vi "Climb Controller.vi"(8 "error in":errorcluster) -> ()   [LabVIEW 2018]
doc: "This VI executes continuously carrying out the current operation and responding to updates or new operations. It will often contain the timing or control code that is difficult to place directly in TeleOp. This VI generally opens all sensors and motors and isolates the rest of the robot code from knowing how the operations are carried out."
uses:
  <vilib>/Rock Robotics/WPI/Framework/Completion Status.ctl
  Climb Setpoints.ctl
  Climb Operations.ctl
  <vilib>/Rock Robotics/SystemInterfaces/DIO/FPGA_DIOChannel.ctl
  <vilib>/Rock Robotics/WPI/ThirdParty/Phoenix-LabVIEW/Motor Controller/Controls/CTRE_Phoenix_MotorControl_FeedbackDevice.ctl
  <vilib>/Rock Robotics/WPI/ThirdParty/REV Robotics/SPARK MAX/Typedef/Spark MAX Control Type.ctl
  <vilib>/Rock Robotics/WPI/ThirdParty/Phoenix-LabVIEW/Motor Controller/Controls/CTRE_Phoenix_MotorControl_ControlMode.ctl
  <vilib>/Rock Robotics/WPI/Switch/WPI_SwitchOpenLimit.vi
  <vilib>/Rock Robotics/WPI/ThirdParty/Phoenix-LabVIEW/Motor Controller/Get/CTRE_Phoenix_MotorController_GetQuadratureData.vi
  <vilib>/Rock Robotics/Network Tables/NT Write Number.vi
  <vilib>/Rock Robotics/Network Tables/NT Write Boolean.vi
  ADIS16448 IMU/ADIS16448_IMU.lvlib
panel:
  in  "Offset Lv 2":dbl=19.75
  in  "Initilization 2":dbl=17.0 format="%#_13g"
  out "IPCed":dbl
  in  "Interactive Values":T1={"Operation"=enum."Read Current", "Setpoint Rhino"=0.0, "Setpoint WHEELS"=0.0, "Roll"=0.0, "Pitch"=0.0, "Reset"=FALSE, "Speedy Tilt"={"Right"=TRUE, "Left"=TRUE}, "Climb"=enum."Level 1-3", "New Pos?"=FALSE, "Defense mode?"=FALSE}
  out "Current\nCmd":string
  in  "Buttons":cluster{"Execute Cmd":bool, "Abort Cmd":bool}
  out "Command Timing":cluster{"Start Time (ms)":u32, "Iterations":i32}
  out "Status":T3
  # "Tip: It may be helpful to observe inputs and sensor values.\nYou may also want to display tuning or debugging controls."
  # "Interactive Command: You may fill in the settings for a command\nand schedule it with the Execute button. You can observe and abort\nany command while fine tuning the code for the controller."
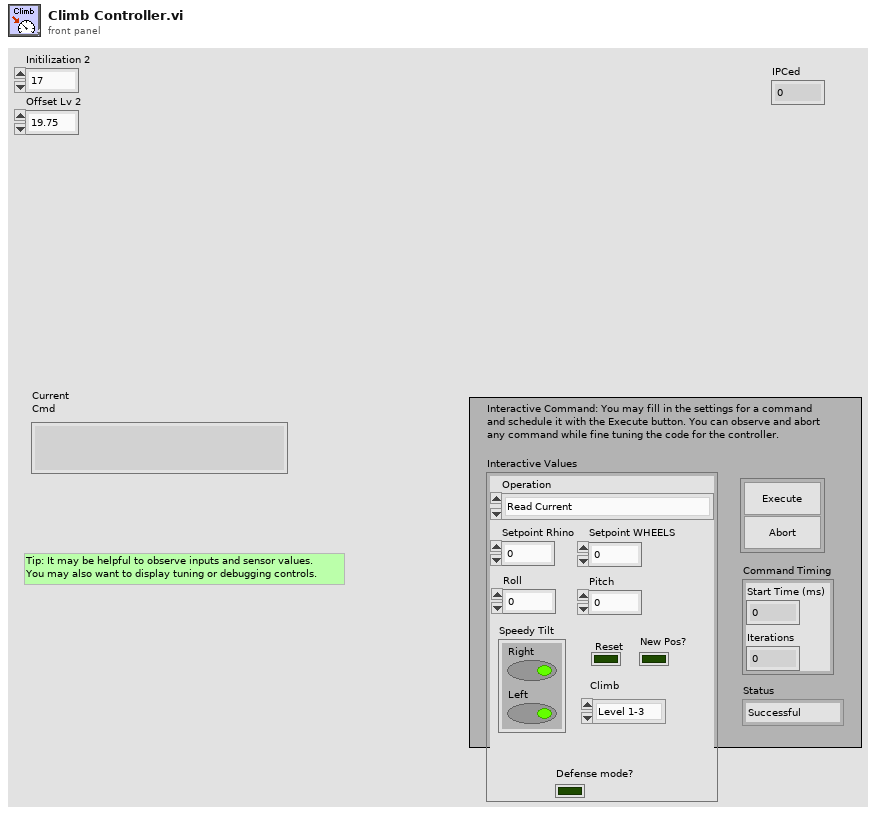
[diagram p1: front panel]
types:
  T1 = typedef "Climb Setpoints.ctl" = cluster{"Operation":T2, "Setpoint Rhino":dbl, "Setpoint WHEELS":dbl, "Roll":dbl, "Pitch":dbl, "Reset":bool, "Speedy Tilt":cluster{"Right":bool, "Left":bool}, "Climb":enum16{"Level 1-3", "Level 1-2", "Level 2-3"}, "New Pos?":bool, "Defense mode?":bool}
  T2 = typedef "Climb Operations.ctl" = enum16{"Reserve", "Read Current", "Immediate", "Ready", "Auto-Climb", "Reset/Turbo-Tilt", "Manual Climb"}
  T3 = typedef "Completion Status.ctl" = enum16{"Successful", "Aborted", "Incomplete"}
  T4 = cluster{"P Gain":dbl, "I Gain":dbl, "D Gain":dbl, "F Gain":dbl, "I Zone":dbl, "Min Output":dbl, "Max Output":dbl}
  T5 = typedef "CTRE_Phoenix_MotorControl_FeedbackDevice.ctl" = i8
  T6 = typedef "FPGA_DIOChannel.ctl" = enum8{"DIO 0", "DIO 1", "DIO 2", "DIO 3", "DIO 4", "DIO 5", "DIO 6", "DIO 7", "DIO 8", "DIO 9", "DIO MXP 0", "DIO MXP 1", "DIO MXP 2", "DIO MXP 3", "DIO MXP 4", "DIO MXP 5", "DIO MXP 6", "DIO MXP 7", "DIO MXP 8", "DIO MXP 9", "DIO MXP 10", "DIO MXP 11", "DIO MXP 12", "DIO MXP 13", "DIO MXP 14", "DIO MXP 15", "SPI Port CS1", "SPI Port CS2", "SPI Port CS3", "SPI Port MISO", "SPI Port MOSI", "Invalid"}
  T7 = typedef "WPI_MotorControlDeviceRef.ctl" = cluster{"DeviceStatus":errorcluster, "Type":T8, "PWM":cluster{"PWM Channel":T9, "DeadBand":T10}, "CAN":cluster{"Device Number":u8, "SetOutput VI Ref":variant, "GetOutput VI Ref":variant, "Enable VI Ref":variant, "Disable VI Ref":variant, "Data":variant}, "Invert":bool, "DIO PWM":cluster{"PWM \"Enable\" Channel":T9, "DIOChannel":T6, "PWM Rate":dbl}}
  T8 = typedef "WPI_MotorControlType.ctl" = enum16{"PWM", "CAN", "DIO PWM"}
  T9 = typedef "FPGA_DIOPWMChannel.ctl" = enum8{"PWM 0", "PWM 1", "PWM 2", "PWM 3", "PWM 4", "PWM 5", "PWM 6", "PWM 7", "PWM 8", "PWM 9", "PWM MXP 0", "PWM MXP 1", "PWM MXP 2", "PWM MXP 3", "PWM MXP 4", "PWM MXP 5", "PWM MXP 6", "PWM MXP 7", "PWM MXP 8", "PWM MXP 9", "Invalid"}
  T10 = typedef "WPI_PWMDeadband.ctl" = cluster{"Name":string, "maxPositivePwm":i32, "minPositivePwm":i32, "centerPwm":i32, "maxNegativePwm":i32, "minNegativePwm":i32, "angularRange":u16}
  T11 = typedef "WPI_SwitchDevRef.ctl" = cluster{"DevStatus":errorcluster, "DIO Channel":T6, "CntIndex":T12, "Normally Closed":bool}
  T12 = typedef "FPGA_CounterCtrSystemIndex.ctl" = enum8{"Ctr 0", "Ctr 1", "Ctr 2", "Ctr 3", "Ctr 4", "Ctr 5", "Ctr 6", "Ctr 7", "Invalid"}
  T13 = typedef "Command Status Info.ctl" = cluster{"Name":string, "Status":T3, "notifier out":T14}
  T14 = typedef "Completion Notifier.ctl" = refnum<notifier>
  T15 = cluster{"Current Command":T1, "Command Timing":cluster{"Start Time (ms)":u32, "Iterations":i32}, "Command Arguments":cluster{"Command Info":T13, "Description":string, "Default Command":T1, "queue out":refnum<queue>, "Subsystem Name":string}}
  T16 = typedef "ADIS16448_IMU.lvlib/ADI_IMU_ADIS16448_IMUDevRef.ctl" = cluster{"DevStatus":errorcluster, "Handle":i32, "SPI Bus":T17, "Device Found":bool, "Device Ready":bool, "Yaw Axis":enum16{"X", "Y", "Z"}, "AHRS Algorithm":enum16{"Complementary", "Madgwick"}, "Serial":u16, "Lot ID 2":u16, "Lot ID 1":u16, "Bytes Per Sample":u16, "Calibrate On Open?":bool}
  T17 = typedef "spi_bus.ctl" = enum16{"SPI On-Board, CS0", "SPI On-Board, CS1", "SPI On-Board, CS2", "SPI On-Board, CS3", "SPI MXP", "Invalid"}
  T18 = typedef "Spark MAX Control Type.ctl" = enum16{"Percent VBus", "Voltage", "Velocity", "Position", "Smart Motion", "Current", "Smart Velocity"}
  T19 = typedef "CTRE_Phoenix_MotorControl_ControlMode.ctl" = u16
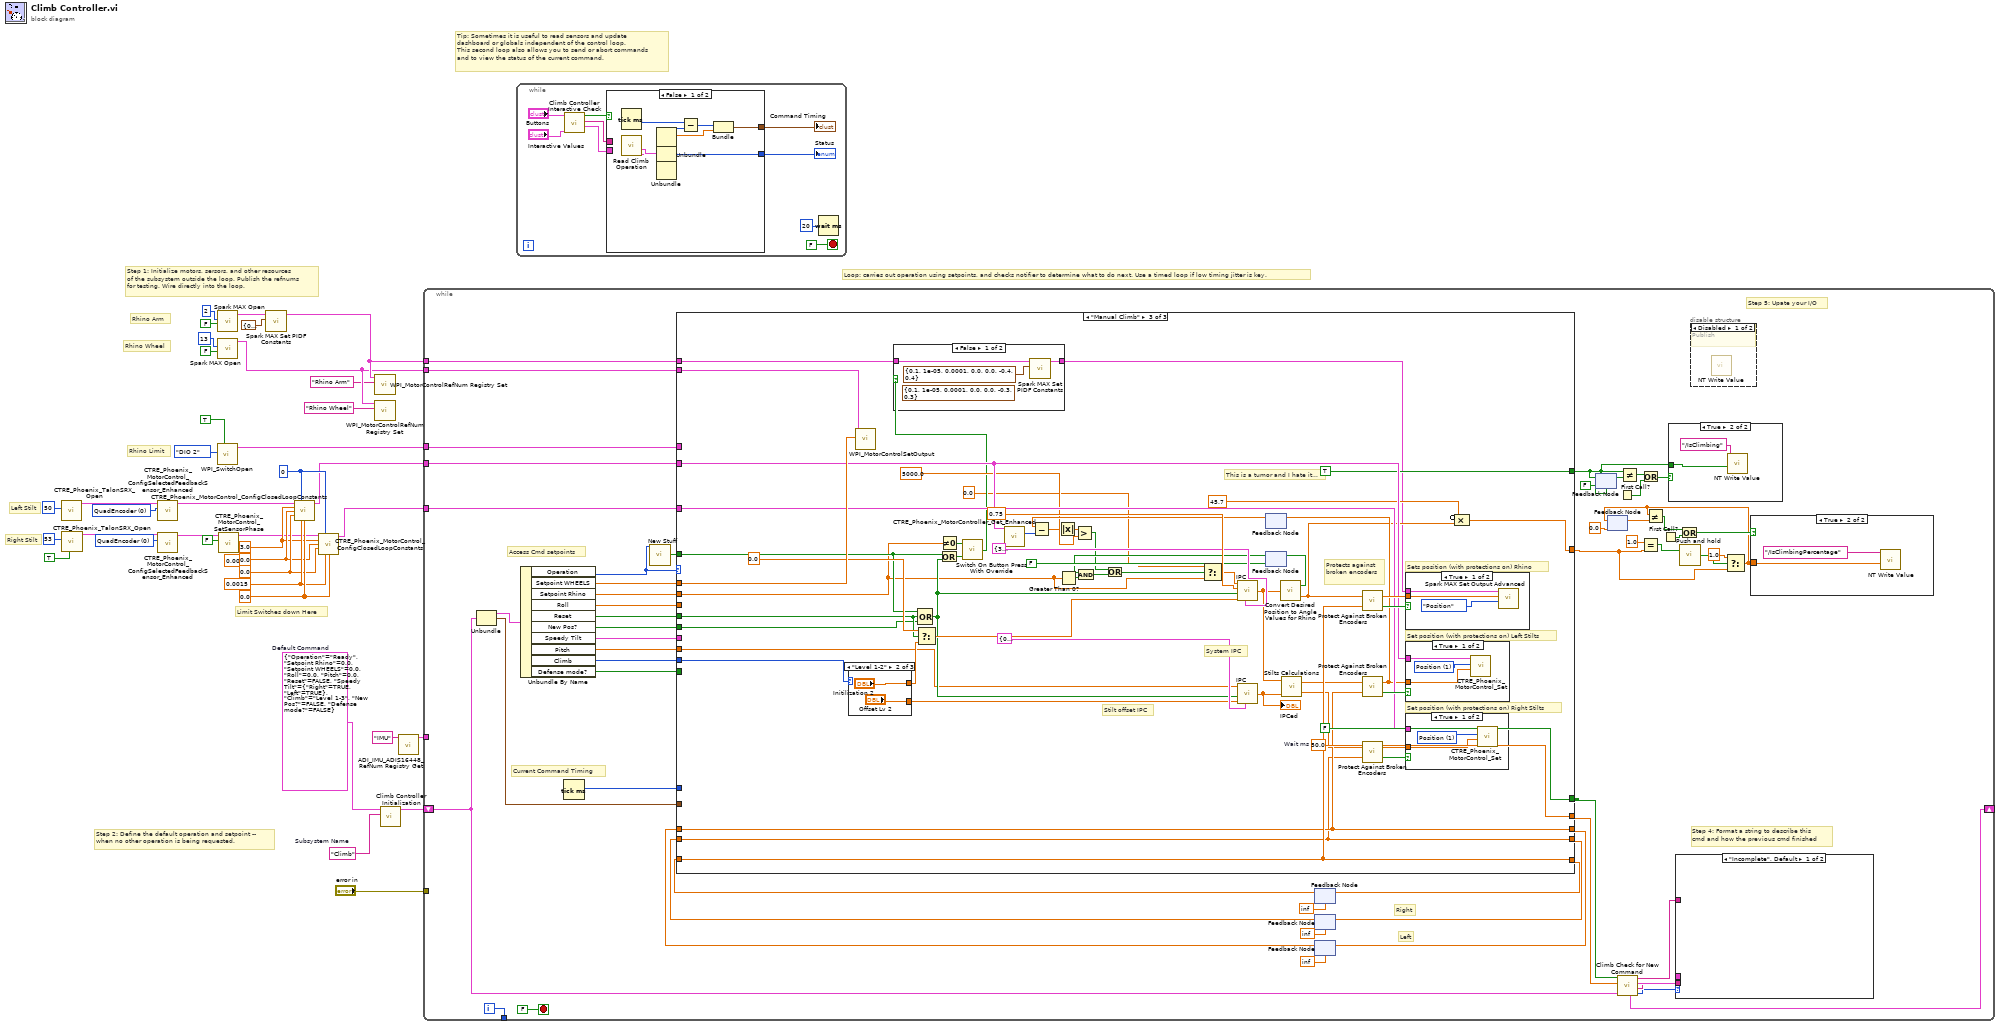
[diagram p0: block diagram]
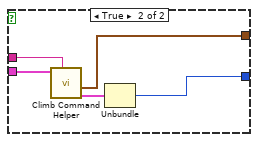
[diagram p2: hidden frame]
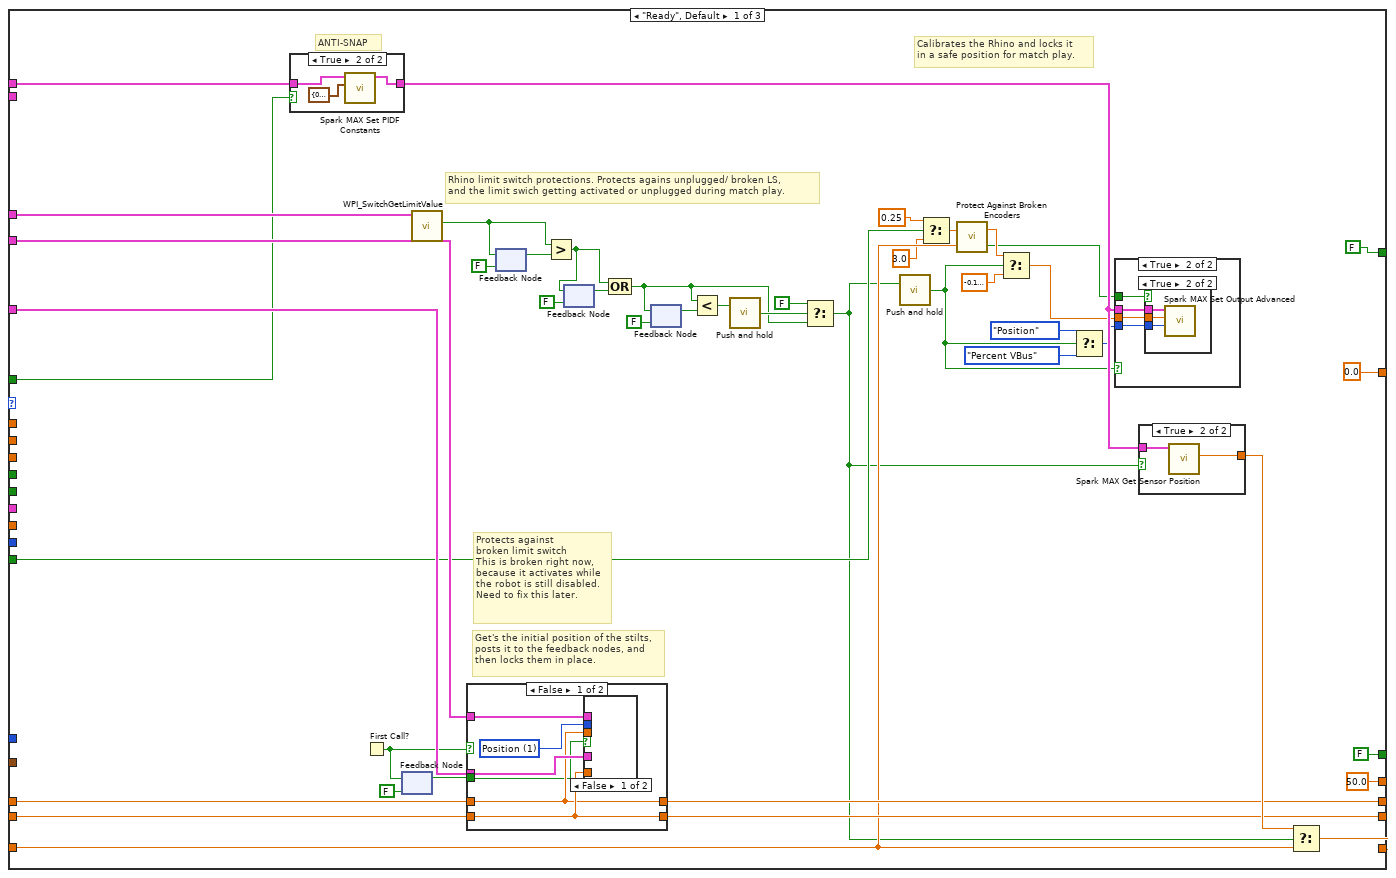
[diagram p5: hidden frame]
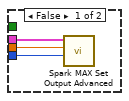
[diagram p6: hidden frame]
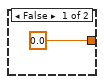
[diagram p9: hidden frame]
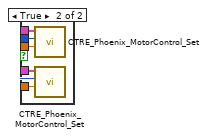
[diagram p10: hidden frame]
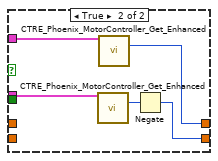
[diagram p11: hidden frame]
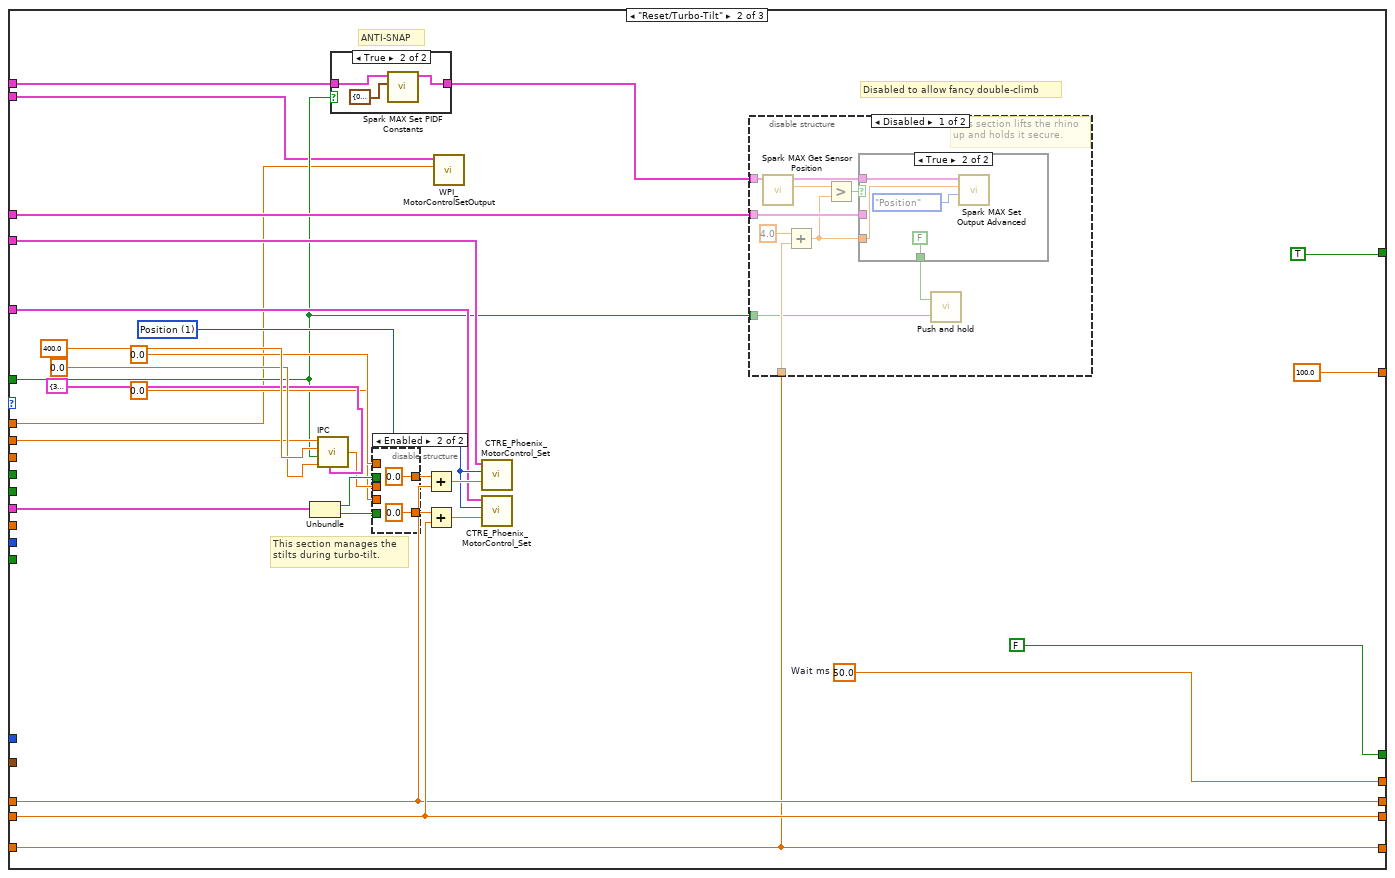
[diagram p12: hidden frame]
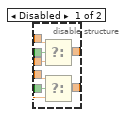
[diagram p13: hidden frame]
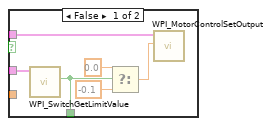
[diagram p14: hidden frame]
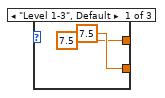
[diagram p17: hidden frame]
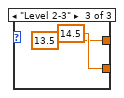
[diagram p18: hidden frame]
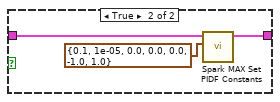
[diagram p19: hidden frame]
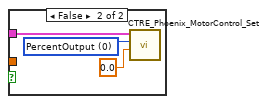
[diagram p20: hidden frame]
diagram:
  (unwired) 0.0001 ("I")
  w16 = 0.0015 ("F")
  w15 = 0.0 ("D")
  w14 = 0.0 ("I")
  w13 = 3.0 ("P")
  w17 = 0.0 ("I Zone")
  w12 = 0 ("slotIdx")
  w24 = T5 0 items=["QuadEncoder"=0, "Analog"=2, "Tachometer"=4, "Pulse Width Encoded Position"=8, "Sensor Sum (S0 + S1)"=9, "Sensor Difference (D0 - D1)"=10, "Remote Source 0"=11, "Remote Source 1"=12, "Software Emulated"=15] ("Feedback Device")
  w25 = T5 0 items=["QuadEncoder"=0, "Analog"=2, "Tachometer"=4, "Pulse Width Encoded Position"=8, "Sensor Sum (S0 + S1)"=9, "Sensor Difference (D0 - D1)"=10, "Remote Source 0"=11, "Remote Source 1"=12, "Software Emulated"=15] ("Feedback Device")
  w5 = T1 {"Operation"=enum."Ready", "Setpoint Rhino"=0.0, "Setpoint WHEELS"=0.0, "Roll"=0.0, "Pitch"=0.0, "Reset"=FALSE, "Speedy Tilt"={"Right"=TRUE, "Left"=TRUE}, "Climb"=enum."Level 1-3", "New Pos?"=FALSE, "Defense mode?"=FALSE}  # Default Command
  w36 = "Climb"  # Subsystem Name
  # "Limit Switches down Here"
  # "Left Stilt"
  # "Rhino Limit"
  # "Right Stilt"
  # "Rhino Wheel"
  # "Rhino Arm"
  # "Tip: Sometimes it is useful to read sensors and update\ndashboard or globals independent of the control loop.\nThis second loop also allows you to send or abort commands\nand to view the status of the current command."
  # "Step 2: Define the default operation and setpoint --\nwhen no other operation is being requested."
  # "Step 1: Initialize motors, sersors, and other resources\nof the subsystem outside the loop. Publish the refnums\nfor testing. Wire directly into the loop."
  # "Loop: carries out operation using setpoints, and checks notifier to determine what to do next. Use a timed loop if low timing jitter is key."
  n1 = call <vilib>:"CTRE_Phoenix_TalonSRX_Open.vi"("Device Number"=u8 50) -> ("CAN Talon SRX Ref"=w23:T7)  [unwired: 9 in, 1 out]
  n2 = call <vilib>:"CTRE_Phoenix_TalonSRX_Open.vi"("Invert"=TRUE, "Device Number"=u8 53) -> ("CAN Talon SRX Ref"=w22:T7)  [unwired: 8 in, 1 out]
  n3 = call <vilib>:"CTRE_Phoenix_MotorControl_ConfigSelectedFeedbackSensor_Enhanced.vi"("Feedback Device"=w24, "PhoenixMotorControlDevRef"=w23) -> ("PhoenixMotorControlDevRef"=w11:T7)  [unwired: 8 in, 1 out]
  n4 = call <vilib>:"CTRE_Phoenix_MotorControl_ConfigSelectedFeedbackSensor_Enhanced.vi"("Feedback Device"=w25, "PhoenixMotorControlDevRef"=w22) -> ("PhoenixMotorControlDevRef"=w21:T7)  [unwired: 8 in, 1 out]
  n5 = call-poly <vilib>:"WPI_SwitchOpen.vi"("Normally Closed"=TRUE, "DIO Channel"=FPGA_DIOChannel."DIO 2") -> ("SwitchDevRef"=w27:T11)  [unwired: 8 in, 1 out]
  n6 = call <vilib>:"Spark MAX Open.vi"("Invert"=FALSE, "Device Number"=u8 2) -> ("MotorControlDeviceRef"=w18:T7)  [unwired: 8 in, 1 out]
  n7 = call <vilib>:"Spark MAX Open.vi"("Invert"=FALSE, "Device Number"=u8 13) -> ("MotorControlDeviceRef"=w3:T7)  [unwired: 8 in, 1 out]
  n8 = call <vilib>:"CTRE_Phoenix_MotorControl_SetSensorPhase.vi"("PhaseSensor"=FALSE, "PhoenixMotorControlDevRef"=w21) -> ("PhoenixMotorControlDevRef"=w10:T7)  [unwired: 8 in, 1 out]
  n9 = call <vilib>:"Spark MAX Set PIDF Constants.vi"("PID Constants"=T4 {"P Gain"=0.1, "I Gain"=1e-05, "D Gain"=0.0, "F Gain"=0.0, "I Zone"=0.0, "Min Output"=-1.0, "Max Output"=1.0}, "MotorControlDeviceRef"=w18) -> ("MotorControlDeviceRef"=w4:T7)  [unwired: 8 in, 1 out]
  n10 = call <vilib>:"CTRE_Phoenix_MotorControl_ConfigClosedLoopConstants.vi"("PhoenixMotorControlDevRef"=w11, "slotIdx"=w12, "P"=w13, "I"=w14, "D"=w15, "F"=w16, "I Zone"=w17) -> ("PhoenixMotorControlDevRef"=w7:T7)  [unwired: 7 in, 1 out]
  n11 = call <vilib>:"CTRE_Phoenix_MotorControl_ConfigClosedLoopConstants.vi"("PhoenixMotorControlDevRef"=w10, "slotIdx"=w12, "P"=w13, "I"=w14, "D"=w15, "F"=w16, "I Zone"=w17) -> ("PhoenixMotorControlDevRef"=w6:T7)  [unwired: 7 in, 1 out]
  n12 = call <vilib>:"WPI_MotorControlRefNum Registry Set.vi"("refnum name"="Rhino Arm", "MotorControlDevRef"=w4) -> ()  [unwired: 8 in, 2 out]
  n13 = call <vilib>:"WPI_MotorControlRefNum Registry Set.vi"("refnum name"="Rhino Wheel", "MotorControlDevRef"=w3) -> ()  [unwired: 8 in, 2 out]
  n14 = call "Climb Controller Initialization.vi"("Subsystem Name"=w36, "Default Command"=w5) -> ("Current Command"=w37:T15)  [unwired: 9 in]
  n15 = call "ADI_IMU_ADIS16448_RefNum Registry Get.vi"("refnum name"="IMU") -> ("ADI IMU DevRef"=w9:T16)  [unwired: 9 in, 1 out]
  n16 = while {
    shift-right: [w88] -> _
    shift-left: w37 -> [w81]
    tunnel: [w92] -> _
    tunnel: "error in" -> [_]
    tunnel: w27 -> [w80]
    tunnel: w4 -> [w76]
    tunnel: w3 -> [w75]
    tunnel: w7 -> [w63]
    tunnel: w6 -> [w62]
    tunnel: w9 -> [_]
    i -> [w92]
    stop <- FALSE stop-if-true
    # "Right"
    # "Left"
    # "Step 5: Upate your I/O"
    # "Step 4: Format a string to describe this\ncmd and how the previous cmd finished"
    # "Current Command Timing"
    # "Access Cmd setpoints"
    n17 = Unbundle(w81) -> ("Current Command"=w91:T1, "Command Timing"=w89:cluster{"Start Time (ms)":u32, "Iterations":i32})  [unwired: 1 out]
    n18 = Unbundle By Name(w91) -> ("Operation"=w61:T2, "Setpoint WHEELS"=w58:dbl, "Setpoint Rhino"=w57:dbl, "Roll"=w68:dbl, "Reset"=w67:bool, "New Pos?"=w66:bool, "Speedy Tilt"=w65:cluster{"Right":bool, "Left":bool}, "Pitch"=w64:dbl, "Climb"=w59:enum16{"Level 1-3", "Level 1-2", "Level 2-3"}, "Defense mode?"=w56:bool)
    n19 = Tick Count (ms)() -> (millisecond timer value=w90:u32)
    n20 = call "New Stuff.vi"("Variant"=w61) -> ("x != y?"=w60:bool)  [unwired: 26 in]
    n21 = feedback #1(inf) -> (w78:dbl)
    n22 = feedback #2(inf) -> (w72:dbl)
    n23 = feedback #3(inf) -> (w71:dbl)
    n24 = case shown="\"Manual Climb\"" w61 {
      tunnel: [50.0 ("Wait ms") w184 w288] -> w86
      tunnel: [FALSE ("Output") FALSE ("Output") FALSE] -> w87
      tunnel: w89 -> [_ _ _]
      tunnel: w57 -> [_ w193 w244]
      tunnel: w90 -> [_ _ _]
      tunnel: w80 -> [w142 w199 _]
      tunnel: [w140 w197 w285] -> w79
      tunnel: w78 -> [w133 w197 w285]
      tunnel: w58 -> [_ w178 w289]
      tunnel: w76 -> [w129 w183 w270]
      tunnel: w75 -> [_ w179 w290]
      tunnel: w63 -> [w135 w195 w275]
      tunnel: w62 -> [w134 w194 w277]
      tunnel: w72 -> [w136 w200 w278]
      tunnel: w71 -> [w137 w198 w282]
      tunnel: [w138 w200 w278] -> w70
      tunnel: [w139 w198 w282] -> w69
      tunnel: w68 -> [_ _ _]
      tunnel: w67 -> [_ _ w247]
      tunnel: w66 -> [_ _ w246]
      tunnel: w65 -> [_ w192 _]
      tunnel: w64 -> [_ _ w245]
      tunnel: w60 -> [w128 w181 w257]
      tunnel: w59 -> [_ _ w248]
      tunnel: w56 -> [w125 _ _]
      tunnel: [FALSE ("Assisted?") TRUE ("Assisted?") TRUE ("Assisted?")] -> w47
      tunnel: [0.0 ("t") 100.0 ("t") w241] -> w41
      frame "Ready", Default {
        # "Rhino limit switch protections. Protects agains unplugged/ broken LS,\nand the limit swich getting activated or unplugged during match play."
        # "Protects against\nbroken limit switch\nThis is broken right now,\nbecause it activates while\nthe robot is still disabled. \nNeed to fix this later."
        # "Calibrates the Rhino and locks it\nin a safe position for match play."
        # "Get's the initial position of the stilts,\nposts it to the feedback nodes, and\nthen locks them in place."
        # "ANTI-SNAP"
        n25 = case shown="True" w128 {
          tunnel: w129 -> [w153 w155]
          tunnel: [w153 w154] -> w124
          frame False {
          }
          frame True {
            n26 = call <vilib>:"Spark MAX Set PIDF Constants.vi"("PID Constants"=T4 {"P Gain"=0.1, "I Gain"=1e-05, "D Gain"=0.0001, "F Gain"=0.0, "I Zone"=0.0, "Min Output"=-0.3, "Max Output"=0.3}, "MotorControlDeviceRef"=w155) -> ("MotorControlDeviceRef"=w154:T7)  [unwired: 8 in, 1 out]
          }
        }
        n27 = First Call?() -> (First Call?: T/F=w132:bool)
        n28 = feedback #4(FALSE ("First Call?: T/F")) -> (w130:bool)
        n29 = feedback-in #4(w132) -> ()
        n30 = call <vilib>:"WPI_SwitchGetLimitValue.vi"("SwitchDevRef"=w142) -> ("Switch Pressed"=w109:bool)  [unwired: 8 in, 2 out]
        n31 = case shown="False" w132 {
          tunnel: w135 -> [w165 w175]
          tunnel: w134 -> [w164 w174]
          tunnel: [w161 w173] -> w139
          tunnel: [w162 w171] -> w138
          tunnel: w137 -> [w161 _]
          tunnel: w136 -> [w162 _]
          tunnel: w130 -> [w160 _]
          frame False {
            w163 = T19 1 items=["PercentOutput"=0, "Position"=1, "Velocity"=2, "Current"=3, "Follower"=5, "MotionProfile"=6, "MotionMagic"=7, "MotionProfileArc"=10, "Disabled"=15] ("Control Mode")
            n32 = case shown="False" w160 {
              tunnel: w165 -> [_ w170]
              tunnel: w164 -> [_ w169]
              tunnel: w163 -> [_ w168]
              tunnel: w162 -> [_ w167]
              tunnel: w161 -> [_ w166]
              frame False {
              }
              frame True {
                n33 = call <vilib>:"CTRE_Phoenix_MotorControl_Set.vi"("Output"=w166, "Control Mode"=w168, "PhoenixMotorControlDevRef"=w170) -> ()  [unwired: 7 in, 2 out]
                n34 = call <vilib>:"CTRE_Phoenix_MotorControl_Set.vi"("Output"=w167, "Control Mode"=w168, "PhoenixMotorControlDevRef"=w169) -> ()  [unwired: 7 in, 2 out]
              }
            }
          }
          frame True {
            n35 = call-poly <vilib>:"CTRE_Phoenix_MotorController_Get_Enhanced.vi"("PhoenixMotorControlDevRef"=w174) -> ("Quadrature Position"=w172:i32)  [unwired: 11 in, 3 out]
            n36 = call-poly <vilib>:"CTRE_Phoenix_MotorController_Get_Enhanced.vi"("PhoenixMotorControlDevRef"=w175) -> ("Quadrature Position"=w173:i32)  [unwired: 11 in, 3 out]
            n37 = Negate(x=w172) -> (-x=w171:i32)
          }
        }
        n38 = feedback-in #5(w109) -> ()
        n39 = feedback #5(FALSE ("Switch Pressed")) -> (w110:bool)
        n40 = Greater?(x=w109, y=w110) -> (0:w106:bool)
        n41 = feedback #6(FALSE ("Switch Pressed")) -> (w105:bool)
        n42 = feedback-in #6(w106) -> ()
        n43 = Compound Arithmetic op=OR(w106, w105) -> (w100:bool)
        n44 = feedback-in #7(w100) -> ()
        n45 = feedback #7(FALSE) -> (w103:bool)
        n46 = Less?(x=w100, y=w103) -> (x < y?=w102:bool)
        n47 = call "Push and hold.vi"("Input"=w102) -> ("Output"=w101:bool)  [unwired: 1 in]
        n48 = Select(t=FALSE, s=w101, f=w100) -> (s? t:f=w98:bool)
        n49 = call "Push and hold.vi"("Input"=w98) -> ("Output"=w111:bool)  [unwired: 1 in]
        n50 = Select(t=0.25, s=w125, f=3.0 ("t")) -> (s? t:f=w114:dbl)
        n51 = call "Protect Against Broken Encoders.vi"("Rhino Offset"=w133, "Output"=w114) -> ("Boolean"=w115:bool, "Numeric"=w118:dbl)
        n52 = Select(t=w118, s=w111, f=-0.10000000000000003) -> (s? t:f=w117:dbl)
        n53 = Select(t=Spark_MAX_Control_Type."Position" ("Control Mode"), s=w111, f=Spark_MAX_Control_Type."Percent VBus" ("Control Mode")) -> (s? t:f=w116:T18)
        n54 = case shown="True" w111 {
          tunnel: w117 -> [w144 w149]
          tunnel: w116 -> [w143 w148]
          tunnel: w124 -> [w145 w147]
          tunnel: w115 -> [_ w146]
          frame False {
            n55 = call <vilib>:"Spark MAX Set Output Advanced.vi"("Control Mode"=w143, "Setpoint"=w144, "MotorControlDevRef"=w145) -> ()  [unwired: 7 in, 2 out]
          }
          frame True {
            n56 = case shown="True" w146 {
              tunnel: w149 -> [_ w152]
              tunnel: w148 -> [_ w151]
              tunnel: w147 -> [_ w150]
              frame False {
              }
              frame True {
                n57 = call <vilib>:"Spark MAX Set Output Advanced.vi"("Control Mode"=w151, "Setpoint"=w152, "MotorControlDevRef"=w150) -> ()  [unwired: 7 in, 2 out]
              }
            }
          }
        }
        n58 = case shown="True" w98 {
          tunnel: [0.0 ("Sensor Position") w159] -> w141
          tunnel: w124 -> [_ w158]
          frame False {
          }
          frame True {
            n59 = call <vilib>:"Spark MAX Get Sensor Position.vi"("MotorControlDevRef in"=w158) -> ("Sensor Position"=w159:dbl)  [unwired: 7 in, 3 out]
          }
        }
        n60 = Select(t=w141, s=w98, f=w133) -> (s? t:f=w140:dbl)
      }
      frame "Reset/Turbo-Tilt" {
        w196 = T19 1 items=["PercentOutput"=0, "Position"=1, "Velocity"=2, "Current"=3, "Follower"=5, "MotionProfile"=6, "MotionMagic"=7, "MotionProfileArc"=10, "Disabled"=15] ("Control Mode")
        w184 = 50.0  # Wait ms
        # "Disabled to allow fancy double-climb"
        # "ANTI-SNAP"
        # "This section manages the\nstilts during turbo-tilt."
        n61 = Unbundle(w192) -> ("Right"=w188:bool, "Left"=w189:bool)
        n62 = call "IPC.vi"("Coerced Values"=cluster{"Max":dbl, "Min":dbl, "Coerce?":bool} {"Max"=32511.0, "Min"=0.0, "Coerce?"=TRUE}, "Initilization"=0.0 ("Multiplier"), "Reset"=w181, "Multiplier"=400.0, "Value"=w193) -> ("IPCed"=w187:dbl)  [unwired: 1 in]
        n63 = case shown="True" w181 {
          tunnel: w183 -> [w235 w238]
          tunnel: [w235 w237] -> w182
          frame False {
          }
          frame True {
            n64 = call <vilib>:"Spark MAX Set PIDF Constants.vi"("PID Constants"=T4 {"P Gain"=0.1, "I Gain"=1e-05, "D Gain"=0.0001, "F Gain"=0.0, "I Zone"=0.0, "Min Output"=-0.3, "Max Output"=0.3}, "MotorControlDeviceRef"=w238) -> ("MotorControlDeviceRef"=w237:T7)  [unwired: 8 in, 1 out]
          }
        }
        n65 = disable-structure shown="Enabled" {
          disable-tunnel: [w212 0.0 ("IPCed")] -> w191
          disable-tunnel: [w211 0.0 ("IPCed")] -> w190
          disable-tunnel: w189 -> [w210 _]
          disable-tunnel: w188 -> [w209 _]
          disable-tunnel: w187 -> [w208 _]
          disable-tunnel: 0.0 ("t") -> [w207 _]
          disable-tunnel: 0.0 ("t") -> [w206 _]
          frame Disabled {
            n66 = Select(t=w207, s=w209, f=w208) -> (s? t:f=w212:dbl)
            n67 = Select(t=w206, s=w210, f=w208) -> (s? t:f=w211:dbl)
          }
          frame Enabled {
          }
        }
        n68 = Add(x=w191, y=w198) -> (x+y=w203:dbl)
        n69 = Add(x=w190, y=w200) -> (x+y=w202:dbl)
        n70 = call <vilib>:"WPI_MotorControlSetOutput.vi"("Output"=w178, "MotorControlDevRef"=w179) -> ()  [unwired: 7 in, 3 out]
        n71 = call <vilib>:"CTRE_Phoenix_MotorControl_Set.vi"("Output"=w203, "Control Mode"=w196, "PhoenixMotorControlDevRef"=w195) -> ()  [unwired: 7 in, 2 out]
        n72 = call <vilib>:"CTRE_Phoenix_MotorControl_Set.vi"("Output"=w202, "Control Mode"=w196, "PhoenixMotorControlDevRef"=w194) -> ()  [unwired: 7 in, 2 out]
        n73 = disable-structure shown="Disabled" {
          disable-tunnel: w199 -> [w223 _]
          disable-tunnel: w197 -> [w219 _]
          disable-tunnel: w182 -> [w217 _]
          disable-tunnel: w181 -> [w215 _]
          frame Disabled {
            # "This section lifts the rhino\nup and holds it secure."
            n74 = call <vilib>:"Spark MAX Get Sensor Position.vi"("MotorControlDevRef in"=w217) -> ("Sensor Position"=w221:dbl, "MotorControlDevRef out"=w224:T7)  [unwired: 7 in, 2 out]
            n75 = Add(x=4.0 ("y"), y=w219) -> (x+y=w218:dbl)
            n76 = Greater?(x=w221, y=w218) -> (0:w222:bool)
            n77 = case shown="True" w222 {
              tunnel: w224 -> [w226 w234]
              tunnel: w223 -> [w227 _]
              tunnel: w218 -> [_ w232]
              tunnel: [w225 FALSE ("Switch Pressed")] -> w216
              frame False {
                n78 = call <vilib>:"WPI_SwitchGetLimitValue.vi"("SwitchDevRef"=w227) -> ("Switch Pressed"=w225:bool)  [unwired: 8 in, 2 out]
                n79 = Select(t=0.0, s=w225, f=-0.1) -> (s? t:f=w230:dbl)
                n80 = call <vilib>:"WPI_MotorControlSetOutput.vi"("Output"=w230, "MotorControlDevRef"=w226) -> ()  [unwired: 7 in, 3 out]
              }
              frame True {
                n81 = call <vilib>:"Spark MAX Set Output Advanced.vi"("Control Mode"=Spark_MAX_Control_Type."Position", "Setpoint"=w232, "MotorControlDevRef"=w234) -> ()  [unwired: 7 in, 2 out]
              }
            }
            n82 = call "Push and hold.vi"("Reset"=w215, "Input"=w216) -> ()  [unwired: 1 out]
          }
          frame Enabled {
          }
        }
      }
      frame "Manual Climb" {
        w288 = 50.0  # Wait ms
        # "This is a tumor and I hate it..."
        # "Protects against\nbroken encoders"
        # "System IPC"
        # "Stilt offset IPC"
        # "Set position (with protections on) Left Stilts"
        # "Set position (with protections on) Right Stilts"
        # "Sets position (with protections on) Rhino"
        n83 = case shown="\"Level 1-2\"" w248 {
          tunnel: [7.5 ("Offset Lv 3") "Offset Lv 2" 14.5 ("Offset Lv 2-3")] -> w267
          tunnel: [7.5 ("Initilization 2") "Initilization 2" 13.5 ("Initilization")] -> w249
          frame "Level 1-3", Default {
          }
          frame "Level 1-2" {
          }
          frame "Level 2-3" {
          }
        }
        n84 = call <vilib>:"WPI_MotorControlSetOutput.vi"("Output"=w289, "MotorControlDevRef"=w290) -> ()  [unwired: 7 in, 3 out]
        n85 = Select(t=0.0, s=w247, f=w249) -> (s? t:f=w264:dbl)
        n86 = Compound Arithmetic op=OR(w257, w247, w246) -> (w263:bool)
        n87 = Not Equal To 0?(x=w244) -> (x != 0?=w268:bool)
        n88 = Or(x=w257, y=w263) -> (x .or. y?=w266:bool)
        n89 = call "Switch On Button Press With Override.vi"("Override False"=w266, "Override True"=w268) -> ("Output"=w269:bool)  [unwired: 1 in]
        n90 = case shown="False" w269 {
          tunnel: w270 -> [w303 w305]
          tunnel: [w302 w304] -> w239
          frame False {
            (unwired) T4 {"P Gain"=0.1, "I Gain"=1e-05, "D Gain"=0.0001, "F Gain"=0.0, "I Zone"=0.0, "Min Output"=-0.3, "Max Output"=0.3} ("PID Constants")
            n91 = call <vilib>:"Spark MAX Set PIDF Constants.vi"("PID Constants"=T4 {"P Gain"=0.1, "I Gain"=1e-05, "D Gain"=0.0001, "F Gain"=0.0, "I Zone"=0.0, "Min Output"=-0.4, "Max Output"=0.4}, "MotorControlDeviceRef"=w303) -> ("MotorControlDeviceRef"=w302:T7)  [unwired: 8 in, 1 out]
          }
          frame True {
            n92 = call <vilib>:"Spark MAX Set PIDF Constants.vi"("PID Constants"=T4 {"P Gain"=0.1, "I Gain"=1e-05, "D Gain"=0.0, "F Gain"=0.0, "I Zone"=0.0, "Min Output"=-1.0, "Max Output"=1.0}, "MotorControlDeviceRef"=w305) -> ("MotorControlDeviceRef"=w304:T7)  [unwired: 8 in, 1 out]
          }
        }
        n93 = call-poly <vilib>:"CTRE_Phoenix_MotorController_Get_Enhanced.vi"("PhoenixMotorControlDevRef"=w275) -> ("Quadrature Position"=w272:i32)  [unwired: 11 in, 3 out]
        n94 = Greater Than 0?(x=w244) -> (x > 0?=w256:bool)
        n95 = call "IPC.vi"("Coerced Values"=cluster{"Max":dbl, "Min":dbl, "Coerce?":bool} {"Max"=0.0, "Min"=0.0, "Coerce?"=FALSE}, "Initilization"=w267, "Reset"=w263, "Value"=w245) -> ("IPCed"=w286:dbl)  [unwired: 2 in]
        "IPCed" <- w286
        n96 = feedback #8() -> (w273:dbl)  [unwired: 1 in]
        n97 = Subtract(x=w273, y=w272) -> (x-y=w259:dbl)
        n98 = Absolute Value(x=w259) -> (abs(x)=w258:dbl)
        n99 = Greater?(x=w258, y=5000.0 ("Stop Climb")) -> (0:w250:bool)
        n100 = feedback #9(FALSE ("Rhino at max position?")) -> (w255:bool)
        n101 = And(x=w255, y=w256) -> (x .and. y?=w251:bool)
        n102 = Or(x=w250, y=w251) -> (x .or. y?=w252:bool)
        n103 = Select(t=0.0, s=w252, f=w244) -> (s? t:f=w253:dbl)
        n104 = call "IPC.vi"("Coerced Values"=cluster{"Max":dbl, "Min":dbl, "Coerce?":bool} {"Max"=32.0, "Min"=0.0, "Coerce?"=TRUE}, "Initilization"=w264, "Reset"=w263, "Multiplier"=0.75, "Value"=w253) -> ("IPCed"=w291:dbl)  [unwired: 1 in]
        n105 = call "Convert Desired Position to Angle Values for Rhino.vi"("Desired Position"=w291) -> ("Rhino at max position?"=w262:bool, "Output"=w240:dbl)
        n106 = feedback-in #9(w262) -> ()
        n107 = call "Stilts Calculations.vi"("Pitch"=w286, "Climb"=w291) -> ("Right"=w279:dbl, "Left"=w274:dbl)  [unwired: 1 in]
        n108 = call "Protect Against Broken Encoders.vi"("Rhino Offset"=w285, "Output"=w240) -> ("Boolean"=w284:bool, "Numeric"=w283:dbl)
        n109 = call "Protect Against Broken Encoders.vi"("Rhino Offset"=w282, "Output"=w274) -> ("Boolean"=w281:bool, "Numeric"=w260:dbl)
        n110 = feedback-in #8(w260) -> ()
        n111 = call "Protect Against Broken Encoders.vi"("Rhino Offset"=w278, "Output"=w279) -> ("Boolean"=w280:bool, "Numeric"=w276:dbl)
        n112 = case shown="True" w284 {
          tunnel: w239 -> [w321 w324]
          tunnel: w283 -> [w319 _]
          frame True {
            n113 = call <vilib>:"Spark MAX Set Output Advanced.vi"("Control Mode"=Spark_MAX_Control_Type."Position", "Setpoint"=w319, "MotorControlDevRef"=w321) -> ()  [unwired: 7 in, 2 out]
          }
          frame False {
            n114 = call <vilib>:"Spark MAX Set Output Advanced.vi"("Control Mode"=Spark_MAX_Control_Type."Percent VBus", "Setpoint"=0.0, "MotorControlDevRef"=w324) -> ()  [unwired: 7 in, 2 out]
          }
        }
        n115 = case shown="True" w281 {
          tunnel: w260 -> [w313 _]
          tunnel: w275 -> [w315 w317]
          frame True {
            w314 = T19 1 items=["PercentOutput"=0, "Position"=1, "Velocity"=2, "Current"=3, "Follower"=5, "MotionProfile"=6, "MotionMagic"=7, "MotionProfileArc"=10, "Disabled"=15] ("Control Mode")
            n116 = call <vilib>:"CTRE_Phoenix_MotorControl_Set.vi"("Output"=w313, "Control Mode"=w314, "PhoenixMotorControlDevRef"=w315) -> ()  [unwired: 7 in, 2 out]
          }
          frame False {
            w316 = T19 0 items=["PercentOutput"=0, "Position"=1, "Velocity"=2, "Current"=3, "Follower"=5, "MotionProfile"=6, "MotionMagic"=7, "MotionProfileArc"=10, "Disabled"=15] ("Control Mode")
            n117 = call <vilib>:"CTRE_Phoenix_MotorControl_Set.vi"("Output"=0.0 ("Setpoint"), "Control Mode"=w316, "PhoenixMotorControlDevRef"=w317) -> ()  [unwired: 7 in, 2 out]
          }
        }
        n118 = case shown="True" w280 {
          tunnel: w276 -> [w307 _]
          tunnel: w277 -> [w308 w311]
          frame True {
            w309 = T19 1 items=["PercentOutput"=0, "Position"=1, "Velocity"=2, "Current"=3, "Follower"=5, "MotionProfile"=6, "MotionMagic"=7, "MotionProfileArc"=10, "Disabled"=15] ("Control Mode")
            n119 = call <vilib>:"CTRE_Phoenix_MotorControl_Set.vi"("Output"=w307, "Control Mode"=w309, "PhoenixMotorControlDevRef"=w308) -> ()  [unwired: 7 in, 2 out]
          }
          frame False {
            w312 = T19 0 items=["PercentOutput"=0, "Position"=1, "Velocity"=2, "Current"=3, "Follower"=5, "MotionProfile"=6, "MotionMagic"=7, "MotionProfileArc"=10, "Disabled"=15] ("Control Mode")
            n120 = call <vilib>:"CTRE_Phoenix_MotorControl_Set.vi"("Output"=0.0 ("Setpoint"), "Control Mode"=w312, "PhoenixMotorControlDevRef"=w311) -> ()  [unwired: 7 in, 2 out]
          }
        }
        n121 = Compound Arithmetic op=MULTIPLY(invert 45.7 ("upper limit"), w240) -> (w241:dbl)
      }
    }
    n122 = feedback-in #1(w79) -> ()
    n123 = feedback-in #2(w70) -> ()
    n124 = feedback-in #3(w69) -> ()
    n125 = feedback #10(FALSE ("Assisted?")) -> (w55:bool)
    n126 = feedback-in #10(w47) -> ()
    n127 = feedback #11(0.0 ("t")) -> (w50:dbl)
    n128 = First Call?() -> (First Call?: T/F=w53:bool)
    n129 = call "Climb Check for New Command.vi"("Current Command"=w81, "Wait time (ms)"=w86, "Finished?"=w87) -> ("Completion"=w82:T3, "Subsystem Name"=w83:string, "Current Command"=w84:T1, "Initial Trace String"=w85:string, "NextCommand"=w88:T15)  [unwired: 4 in]
    n130 = Not Equal?(x=w47, y=w55) -> (x != y?=w52:bool)
    n131 = Or(x=w52, y=w53) -> (x .or. y?=w51:bool)
    n132 = Equal?(x=1.0, y=w41) -> (x = y?=w44:bool)
    n133 = First Call?() -> (First Call?: T/F=w48:bool)
    n134 = case shown="True" w51 {
      tunnel: w47 -> [_ w96]
      frame False {
      }
      frame True {
        n135 = call-poly <vilib>:"NT Write Value.vi"("Boolean"=w96, "Name"="/IsClimbing") -> ()  [unwired: 9 in, 1 out]
      }
    }
    n136 = case shown="\"Incomplete\", Default" w82 {
      selector: w82 -> [_ w332]
      tunnel: w85 -> [_ w328]
      tunnel: w84 -> [_ w329]
      tunnel: w83 -> [_ w325]
      frame "Incomplete", Default {
        # "Continuing current command"
      }
      frame "Successful", "Aborted" {
        # "Finished? &\nWait Time"
        # "Report and setup for next command"
        n137 = Unbundle By Name(w329) -> ("Operation"=w331:T2, "Setpoint Rhino"=w326:dbl)
        n138 = Format Into String(format string="S %.1f, D %f", initial string=w328, w331, w326) -> (resulting string=w327:string)  [unwired: 1 in, 1 out]
        "Current\nCmd" <- w327
        n139 = call <vilib>:"Trace Results.vi"("Status of previous command"=w332, "Description"=w327, "Subsystem"=w325) -> ()  [unwired: 9 in]
      }
    }
    n140 = call "Push and hold.vi"("Input"=w44) -> ("Output"=w42:bool)  [unwired: 1 in]
    n141 = disable-structure shown="Disabled" {
      frame Disabled {
        # "Publish"
        n142 = call-poly <vilib>:"NT Write Value.vi"() -> ()  [unwired: 11 in, 1 out]
      }
      frame Enabled {
      }
    }
    n143 = Select(t=1.0, s=w42, f=w41) -> (s? t:f=w39:dbl)
    n144 = feedback-in #11(w39) -> ()
    n145 = Not Equal?(x=w39, y=w50) -> (x != y?=w45:bool)
    n146 = Or(x=w45, y=w48) -> (x .or. y?=w46:bool)
    n147 = case shown="True" w46 {
      tunnel: w39 -> [_ w94]
      frame False {
      }
      frame True {
        n148 = call-poly <vilib>:"NT Write Value.vi"("Numeric"=w94, "Name"="/IsClimbingPercentage") -> ()  [unwired: 9 in, 1 out]
      }
    }
  }
  n149 = while {
    stop <- FALSE stop-if-true
    n150 = call "Climb Controller Interactive Check.vi"("Interactive Command in"="Interactive Values", "Buttons"="Buttons") -> ("Interactive Command out"=w336:T1, "Trace String"=w337:string, "Schedule"=w338:bool)  [unwired: 7 in]
    n151 = case shown="False" w338 {
      tunnel: [w349 w354] -> w335
      tunnel: w336 -> [_ w352]
      tunnel: [w345 w350] -> w334
      tunnel: w337 -> [_ w353]
      frame False {
        n152 = Tick Count (ms)() -> (millisecond timer value=w344:u32)
        n153 = call "Read Climb Operation.vi"() -> ("Command Info"=w342:T13, "SubSystem Data"=w343:T1)  [unwired: 9 in, 1 out]
        n154 = Unbundle(w343) -> ("Operation"=w348:T2, "Setpoint Rhino"=w346:dbl)  [unwired: 8 out]
        n155 = Unbundle(w342) -> ("Status"=w349:T3)  [unwired: 2 out]
        n156 = Subtract(x=w344, y=w348) -> (x-y=w347:u32)
        n157 = Bundle(w347, "Setpoint Rhino"=w346) -> (w345:cluster{u32, "Setpoint Rhino":dbl})  [unwired: 1 in]
      }
      frame True {
        n158 = call "Climb Command Helper.vi"("Description"=w353, "SubSystem Data"=w352) -> ("Command Info Out"=w351:T13, "Command Timing"=w350:cluster{"Start Time (ms)":u32, "Iterations":i32})  [unwired: 7 in, 1 out]
        n159 = Unbundle(w351) -> ("Status"=w354:T3)  [unwired: 2 out]
      }
    }
    "Status" <- w335
    "Command Timing" <- w334
    n160 = Wait (ms)(milliseconds to wait=u32 20) -> ()  [unwired: 1 out]
  }
